vi "Stoichiometric Calculate.vi"(11 "Stoic Parameter":T1) -> (2 "Air Flow":dbl, 3 "H2 Flow":dbl)   [LabVIEW 2020]
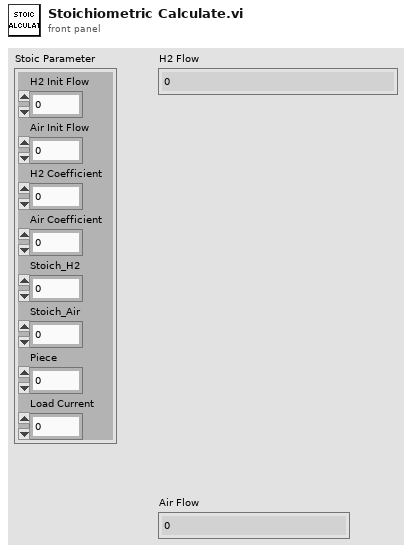
[diagram p1: front panel]
types:
  T1 = cluster{"H2 Init Flow":dbl, "Air Init Flow":dbl, "H2 Coefficient":dbl, "Air Coefficient":dbl, "Stoich_H2":dbl, "Stoich_Air":dbl, "Piece":u32, "Load Current":dbl}
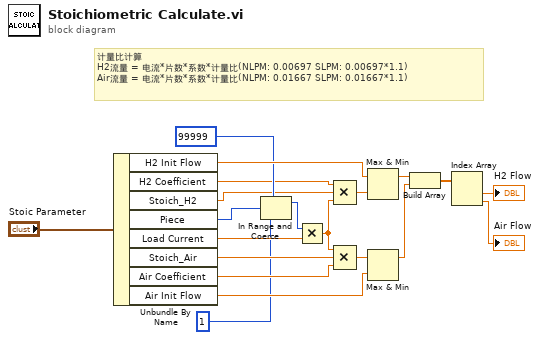
[diagram p0: block diagram]
diagram:
  # "计量比计算\nH2流量 = 电流*片数*系数*计量比(NLPM: 0.00697 SLPM: 0.00697*1.1)\nAir流量 = 电流*片数*系数*计量比(NLPM: 0.01667 SLPM: 0.01667*1.1)"
  n1 = Unbundle By Name("Stoic Parameter") -> ("H2 Init Flow"=w12:dbl, "H2 Coefficient"=w5:dbl, "Stoich_H2"=w6:dbl, "Piece"=w7:u32, "Load Current"=w20:dbl, "Stoich_Air"=w10:dbl, "Air Coefficient"=w11:dbl, "Air Init Flow"=w15:dbl)
  n2 = In Range and Coerce(upper limit=u32 99999 ("上限"), x=w7, lower limit=u32 1 ("下限")) -> (coerced(x)=w19:u32)  [unwired: 1 out]
  n3 = Multiply(x=w19, y=w20) -> (x*y=w18:dbl)
  n4 = Compound Arithmetic op=MULTIPLY(w5, w6, w18) -> (w13:dbl)
  n5 = Compound Arithmetic op=MULTIPLY(w18, w10, w11) -> (w14:dbl)
  n6 = Max & Min(x=w12, y=w13) -> (max(x,y)=w16:dbl)  [unwired: 1 out]
  n7 = Max & Min(x=w14, y=w15) -> (max(x,y)=w17:dbl)  [unwired: 1 out]
  n8 = Build Array(w16, w17) -> (w3:dbl[])
  n9 = Index Array(array=w3) -> (element #1=→"H2 Flow":dbl, element #2=→"Air Flow":dbl)  [unwired: 2 in]
